vi "VarArrayPROCESS.vi"(6 "Process Select In":T1, 8 "Error In":errorcluster, 9 "Select Array In":variant[](array[variant]), 10 "Index Array In":i32[](array[numeric]), 11 "Array In":variant[](array[variant])) -> (0 "Error Out":errorcluster, 1 "Selected Array Out":variant[](array[variant]), 2 "Index Array Out":i32[](array[numeric]), 3 "Array Out":variant[](array[variant]), 4 "First Item Out":variant)   [LabVIEW 2015]
uses:
  TypeDefs_Utility/ENUM_VarArray_Process select.ctl
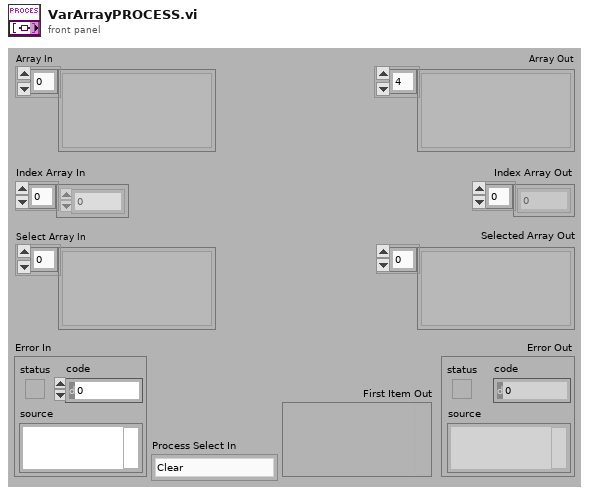
[diagram p1: front panel]
types:
  T1 = typedef "ENUM_VarArray_Process select.ctl" = enum16{"Clear", "Add to beginning", "Add to End", "Replace", "Read", "Find and Remove", "Find", "Insert", "Delete", "Get First Items", "Remove first Item", "Get Item", "No Action", "Replace Items", "Find and Replace Items"}
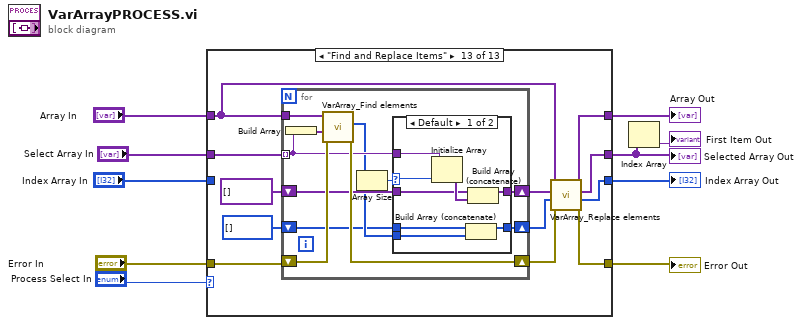
[diagram p0: block diagram]
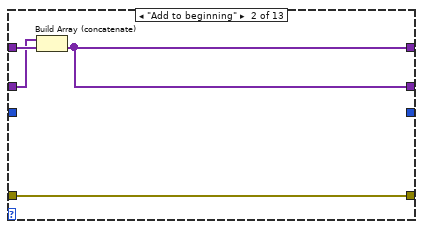
[diagram p3: hidden frame]
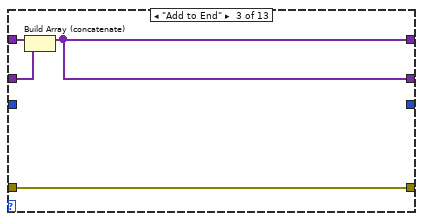
[diagram p4: hidden frame]
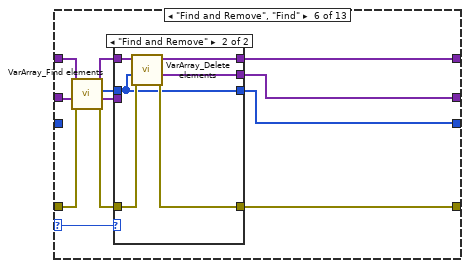
[diagram p7: hidden frame]
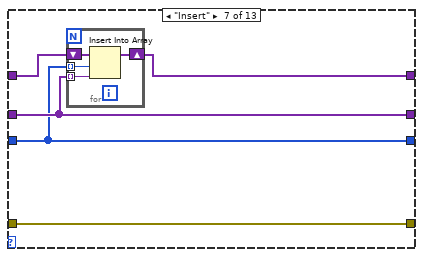
[diagram p9: hidden frame]
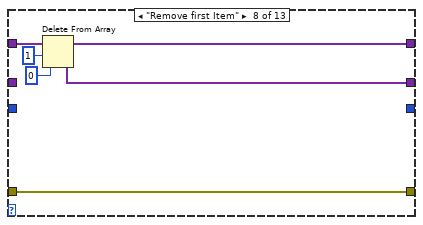
[diagram p10: hidden frame]
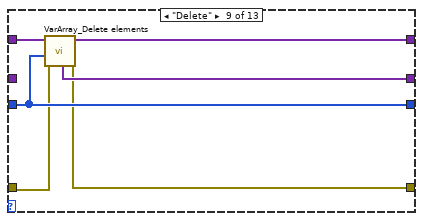
[diagram p11: hidden frame]
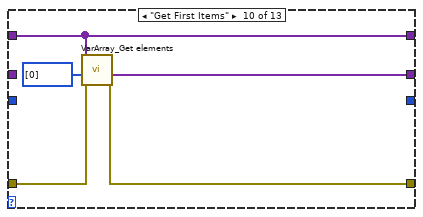
[diagram p12: hidden frame]
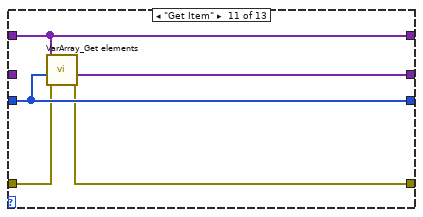
[diagram p13: hidden frame]
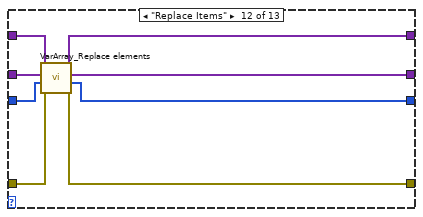
[diagram p14: hidden frame]
diagram:
  n1 = case shown="\"Find and Replace Items\"" "Process Select In" {
    selector: "Process Select In" -> [_ _ _ _ _ w34 _ _ _ _ _ _ _]
    tunnel: "Array In" -> [_ w15 w19 _ w23 w35 w50 w60 w66 w71 w76 w84 w87]
    tunnel: [_ w13 w17 w21 w23 w32 w49 w59 w65 w71 w76 w83 w96] -> w8
    tunnel: "Select Array In" -> [_ w14 w18 w21 _ w30 w48 _ _ _ _ w78 w90]
    tunnel: "Index Array In" -> [_ _ _ _ _ _ w47 _ w63 _ w74 w80 _]
    tunnel: [_ _ _ _ _ w24 w47 _ w63 _ w74 w79 w91] -> w6
    tunnel: [_ w13 w17 w21 w23 w31 w48 w56 w64 w69 w75 w77 w92] -> w4
    tunnel: "Error In" -> [w11 w12 w16 w20 w22 w27 w46 w55 w62 w68 w73 w82 w94]
    tunnel: [w11 w12 w16 w20 w22 w29 w46 w55 w61 w67 w72 w81 w95] -> w1
    frame "Clear" {
    }
    frame "Add to beginning" {
      n2 = Build Array (concatenate)(w14, w15) -> (w13:variant[])
    }
    frame "Add to End" {
      n3 = Build Array (concatenate)(w19, w18) -> (w17:variant[])
    }
    frame "Replace" {
    }
    frame "Read", "No Action" {
    }
    frame "Find and Remove", "Find" {
      n4 = call "VarArray_Find elements.vi"("Error In"=w27, "Select Array In"=w30, "Array In"=w35) -> ("Error Out"=w26:errorcluster, "Selected Array Out"=w28:variant[], "Index Array Out"=w25:i32[], "Array Out"=w33:variant[])  [unwired: 5 in]
      n5 = case shown="\"Find and Remove\"" w34 {
        tunnel: w25 -> [w36 w40]
        tunnel: w33 -> [w39 w45]
        tunnel: [w39 w44] -> w32
        tunnel: [w38 w43] -> w31
        tunnel: w28 -> [w38 _]
        tunnel: w26 -> [w37 w42]
        tunnel: [w37 w41] -> w29
        tunnel: [w36 w40] -> w24
        frame Default {
        }
        frame "Find and Remove" {
          n6 = call "VarArray_Delete elements.vi"("Error In"=w42, "Index Array In"=w40, "Array In"=w45) -> ("Error Out"=w41:errorcluster, "Deleted Elements Out"=w43:variant[], "Array Out"=w44:variant[])  [unwired: 6 in]
        }
      }
    }
    frame "Insert" {
      n7 = for {
        tunnel: w48 -> [w52] mode=indexing
        tunnel: w47 -> [w51] mode=indexing
        shift-right: [w53] -> w49
        shift-left: w50 -> [w54]
        n8 = Insert Into Array(array=w54, index=w51, new element=w52) -> (w53:variant[])
      }
    }
    frame "Remove first Item" {
      n9 = Delete From Array(array=w60, length=1, index=0) -> (deleted portion=w56:variant[], array with subset deleted=w59:variant[])
    }
    frame "Delete" {
      n10 = call "VarArray_Delete elements.vi"("Error In"=w62, "Index Array In"=w63, "Array In"=w66) -> ("Error Out"=w61:errorcluster, "Deleted Elements Out"=w64:variant[], "Array Out"=w65:variant[])  [unwired: 6 in]
    }
    frame "Get First Items" {
      n11 = call "VarArray_Get elements.vi"("Error In"=w68, "Index Array In"=i32[] [0] ("Secondary array in"), "Array In In"=w71) -> ("Error Out"=w67:errorcluster, "Selected Array Out"=w69:variant[])  [unwired: 7 in]
    }
    frame "Get Item" {
      n12 = call "VarArray_Get elements.vi"("Error In"=w73, "Index Array In"=w74, "Array In In"=w76) -> ("Error Out"=w72:errorcluster, "Selected Array Out"=w75:variant[])  [unwired: 7 in]
    }
    frame "Replace Items" {
      n13 = call "VarArray_Replace elements.vi"("Error In"=w82, "Index Array In"=w80, "Replace Array In"=w78, "Array In In In"=w84) -> ("Error Out"=w81:errorcluster, "Replaced Indexs Out"=w79:i32[], "Replaced Data Out"=w77:variant[], "Array Out"=w83:variant[])  [unwired: 4 in]
    }
    frame "Find and Replace Items" {
      n14 = for {
        tunnel: w90 -> [w102] mode=indexing
        tunnel: w87 -> [w105]
        shift-right: [w101] -> w85
        shift-left: variant[] [] -> [w100]
        shift-right: [w98] -> w86
        shift-left: i32[] [] -> [w97]
        shift-right: [w106] -> w93
        shift-left: w94 -> [w107]
        n15 = Build Array(w102) -> (w104:variant[])
        n16 = call "VarArray_Find elements.vi"("Error In"=w107, "Select Array In"=w104, "Array In"=w105) -> ("Error Out"=w106:errorcluster, "Index Array Out"=w99:i32[])  [unwired: 5 in, 2 out]
        n17 = Array Size(array=w99) -> (size(s)=w103:i32)
        n18 = case shown="Default" w103 {
          selector: w103 -> [w115 _]
          tunnel: w102 -> [w114 _]
          tunnel: [w112 w117] -> w101
          tunnel: w100 -> [w111 w117]
          tunnel: w99 -> [w110 _]
          tunnel: [w109 w116] -> w98
          tunnel: w97 -> [w108 w116]
          frame Default {
            n19 = Initialize Array(w114, w115) -> (w113:variant[])
            n20 = Build Array (concatenate)(w108, w110) -> (w109:i32[])
            n21 = Build Array (concatenate)(w111, w113) -> (w112:variant[])
          }
          frame 0 {
          }
        }
      }
      n22 = call "VarArray_Replace elements.vi"("Error In"=w93, "Index Array In"=w86, "Replace Array In"=w85, "Array In In In"=w87) -> ("Error Out"=w95:errorcluster, "Replaced Indexs Out"=w91:i32[], "Replaced Data Out"=w92:variant[], "Array Out"=w96:variant[])  [unwired: 4 in]
    }
  }
  "Array Out" <- w8
  "Index Array Out" <- w6
  "Selected Array Out" <- w4
  "Error Out" <- w1
  n23 = Index Array(array=w4) -> (element=→"First Item Out":variant)  [unwired: 1 in]
